vi "Deep Learning Object Detection - Overlay Results.vi"(7 "Image Scaling":cluster{"X":dbl, "Y":dbl}, 8 "error in (no error)":errorcluster, 9 "Minimum Score Threshold":sgl=0.5, 10 "Detected Objects":T3[](array[typedef]) {"Bounding Box"."y" format="%.2f"; "Bounding Box"."x" format="%.2f"}, 11 "Image In":T2) -> (0 "error out":errorcluster, 3 "Image Out":T2)   [LabVIEW 2020]
uses:
  <vilib>/vision/Deep Learning.llb/IMAQ DL Model Objects.ctl
  <vilib>/vision/Image Controls.llb/IMAQ Image.ctl
panel:
  in  "Font":T1={"Desired Font (Application)"=enum."User-specified Font", "[User-specified Font]"={"Font Name"="Segoe UI", "Size"=24, "Strikeout?"=FALSE, "Italic?"=FALSE, "Underline?"=FALSE, "Outline?"=FALSE, "Shadow?"=FALSE, "Bold?"=TRUE, "Rotation Angle"=0.0}, "Horizontal Alignment"=0, "Vertical Alignment"=0} {"Vertical Alignment" items=["Bottom", "Top", "Baseline"]; "Horizontal Alignment" items=["Left", "Center", "Right"]; "[User-specified Font]"."Rotation Angle" format="%.2f"}
  in  "Color Box":u32(colorbox)=16711680
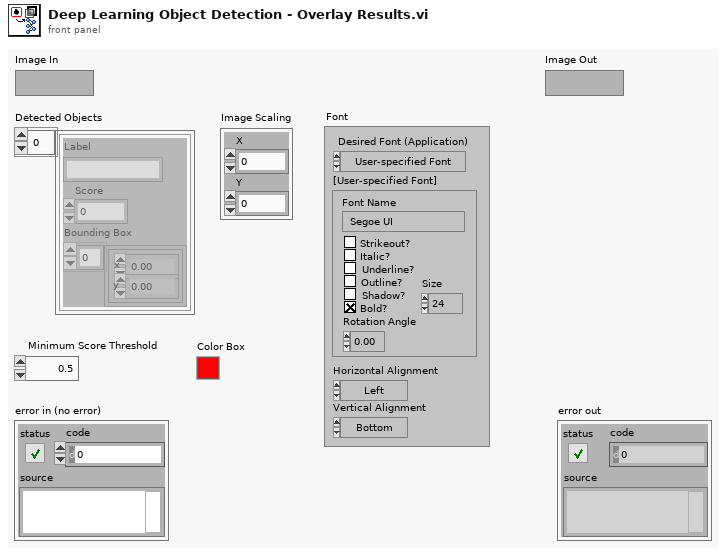
[diagram p1: front panel]
types:
  T1 = cluster{"Desired Font (Application)":enum16{"User-specified Font", "Application Font", "System Font", "Dialog Font"}, "[User-specified Font]":cluster{"Font Name":string, "Size":i16, "Strikeout?":bool, "Italic?":bool, "Underline?":bool, "Outline?":bool, "Shadow?":bool, "Bold?":bool, "Rotation Angle":dbl}, "Horizontal Alignment":i16, "Vertical Alignment":i16}
  T2 = typedef "IMAQ Image.ctl" = refnum<image>
  T3 = typedef "IMAQ DL Model Objects.ctl" = cluster{"Label":string, "Score":sgl, "Bounding Box":cluster{"x":sgl, "y":sgl}[]}
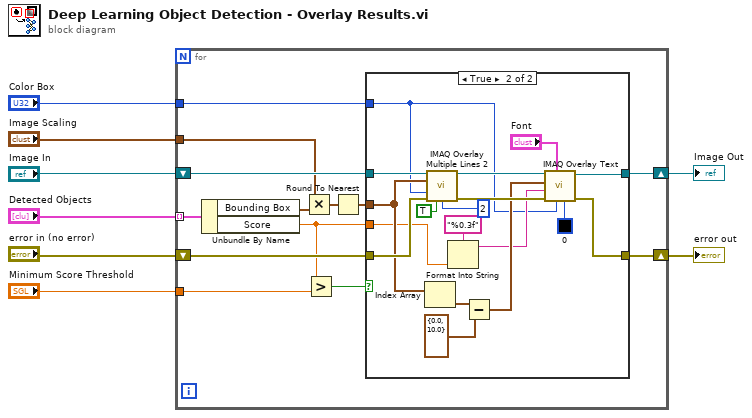
[diagram p0: block diagram]
diagram:
  n1 = for {
    tunnel: "Detected Objects" -> [w21] mode=indexing
    shift-right: [w17] -> w3
    shift-left: "error in (no error)" -> [w18]
    shift-right: [w16] -> w7
    shift-left: "Image In" -> [w20]
    tunnel: "Minimum Score Threshold" -> [w15]
    tunnel: "Color Box" -> [w13]
    tunnel: "Image Scaling" -> [w11]
    n2 = Unbundle By Name(w21) -> ("Bounding Box"=w12:cluster{"x":sgl, "y":sgl}[], "Score"=w14:sgl)
    n3 = Multiply(x=w11, y=w12) -> (x*y=w10:cluster{dbl, dbl}[])
    n4 = Greater?(x=w14, y=w15) -> (0:w19:bool)
    n5 = Round To Nearest(number=w10) -> (nearest integer value=w9:cluster{dbl, dbl}[])
    n6 = case shown="True" w19 {
      tunnel: w20 -> [w22 w41]
      tunnel: w9 -> [_ w35]
      tunnel: w18 -> [w23 w40]
      tunnel: [w23 w36] -> w17
      tunnel: [w22 w37] -> w16
      tunnel: w14 -> [_ w31]
      tunnel: w13 -> [_ w28]
      frame False {
      }
      frame True {
        n7 = Index Array(array=w35) -> (element=w34:cluster{dbl, dbl})  [unwired: 1 in]
        n8 = call "IMAQ Overlay Multiple Lines 2"("Image"=w41, "Line End Points"=w35, "Color"=w28, "error in (no error)"=w40, "Maintain Width?"=TRUE, "Width"=u32 2) -> ("Image Out"=w39:T2, "error out"=w38:errorcluster)  [unwired: 8 in]
        n9 = Format Into String(format string="%0.3f", w31) -> (resulting string=w29:string)  [unwired: 2 in, 1 out]
        n10 = Subtract(x=w34, y=cluster{"X":dbl, "Y":dbl} {"X"=0.0, "Y"=10.0}) -> (x-y=w32:cluster{dbl, dbl})
        n11 = call "IMAQ Overlay Text"("BG Color (Transparent)"=u32 0, "Text Color (black)"=w28, "Font, Size & Style"="Font", "error in (no error)"=w38, "String"=w29, "Origin"=w32, "Image"=w39) -> ("error out"=w36:errorcluster, "Image Out"=w37:T2)  [unwired: 3 in]
      }
    }
  }
  "Image Out" <- w7
  "error out" <- w3
